vi "GetVersion.vi"(6 "error in":errorcluster, 9 "connection ID":refnum<k5>) -> (0 "error out":errorcluster, 3 "connection ID out":refnum<k5>, 4 "Version":T1)   [LabVIEW 2014, in "Raspberry Pi Compatible Compiler for LabVIEW.lvlib" / "RasPiDownloader.lvlib"]
uses:
  RasPiDownloader.lvlib
  RuntimeVersion.ctl
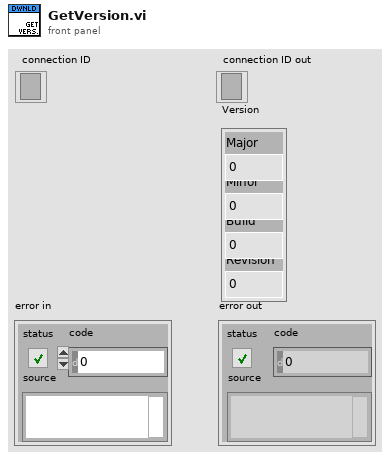
[diagram p1: front panel]
types:
  T1 = typedef "Raspberry Pi Compatible Compiler for LabVIEW.lvlib/RasPiDownloader.lvlib/RuntimeVersion.ctl" = cluster{"Major":i32, "Minor":i32, "Build":i32, "Revision":i32}
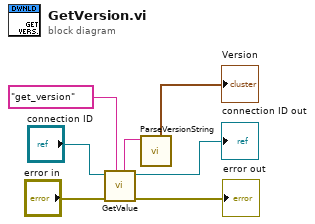
[diagram p0: block diagram]
diagram:
  n1 = call "GetValue.vi"("cmd"="get_version", "error in"="error in", "connection ID"="connection ID") -> ("error out"=→"error out":errorcluster, "connection ID out"=→"connection ID out":refnum<k5>, "value"=w7:string)  [unwired: 4 in]
  n2 = call "ParseVersionString.vi"("version string"=w7) -> ("Version"=→"Version":T1)  [unwired: 7 in, 1 out]
